vi "WMI Get Battery Status.vi"() -> (0 "Discharging?":bool, 1 "estRT":i32, 2 "estCharge":u8, 3 "Status":string)   [LabVIEW 2013]
doc: "Use the WMI to return the battery status, including the estimated battery life remaining and the time until the battery is fully discharged.\n\nInformation regarding the WMI battery class may be found at http://msdn.microsoft.com/en-us/library/aa394074%28v=vs.85%29.aspx."
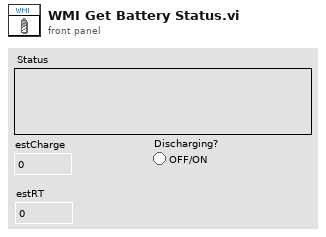
[diagram p1: front panel]
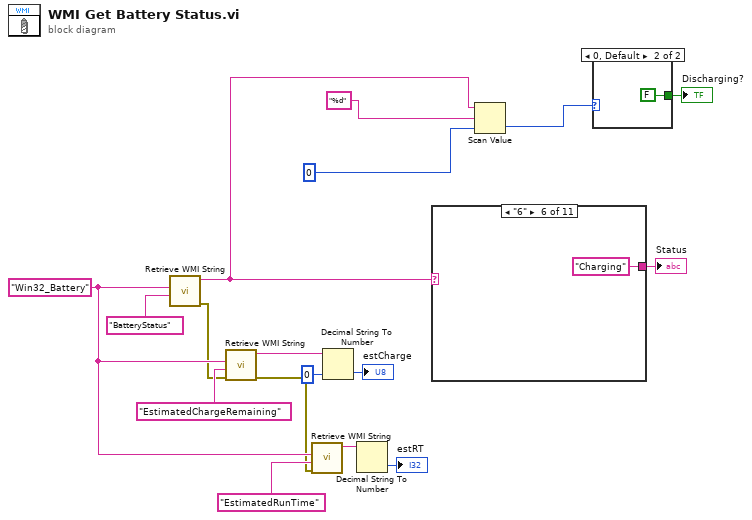
[diagram p0: block diagram]
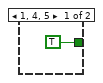
[diagram p2: hidden frame]
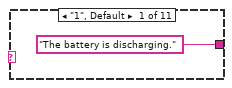
[diagram p3: hidden frame]
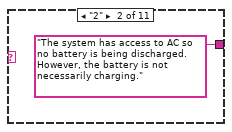
[diagram p4: hidden frame]
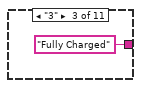
[diagram p5: hidden frame]
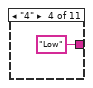
[diagram p6: hidden frame]
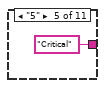
[diagram p7: hidden frame]
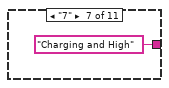
[diagram p8: hidden frame]
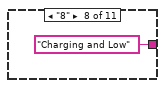
[diagram p9: hidden frame]
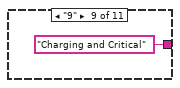
[diagram p10: hidden frame]
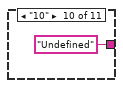
[diagram p11: hidden frame]
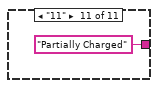
[diagram p12: hidden frame]
diagram:
  w15 = "Win32_Battery" ("wmiClass")
  n1 = call "Retrieve WMI String.vi"("wmiProperty"="BatteryStatus", "wmiClass"=w15) -> ("Error Out"=w7:errorcluster, "LastValue"=w2:string)  [unwired: 7 in, 1 out]
  n2 = call "Retrieve WMI String.vi"("error in"=w7, "wmiProperty"="EstimatedChargeRemaining", "wmiClass"=w15) -> ("Error Out"=w8:errorcluster, "LastValue"=w11:string)  [unwired: 6 in, 1 out]
  n3 = call "Retrieve WMI String.vi"("error in"=w8, "wmiProperty"="EstimatedRunTime", "wmiClass"=w15) -> ("LastValue"=w13:string)  [unwired: 6 in, 2 out]
  n4 = Decimal String To Number(string=w11, default (0L)=u8 0 ("default (0 I32)")) -> (number=→"estCharge":u8)  [unwired: 1 in, 1 out]
  n5 = Decimal String To Number(string=w13) -> (number=→"estRT":i32)  [unwired: 2 in, 1 out]
  n6 = case shown="\"6\"" w2 {
    tunnel: ["The battery is discharging." "The system has access to AC so no battery is being discharged. However, the battery is not necessarily charging." "Fully Charged" "Low" "Critical" "Charging" "Charging and High" "Charging and Low" "Charging and Critical" "Undefined" "Partially Charged"] -> w9
    frame "1", Default {
    }
    frame "2" {
    }
    frame "3" {
    }
    frame "4" {
    }
    frame "5" {
    }
    frame "6" {
    }
    frame "7" {
    }
    frame "8" {
    }
    frame "9" {
    }
    frame "10" {
    }
    frame "11" {
    }
  }
  "Status" <- w9
  n7 = Scan Value(string=w2, format string="%d", default (0 dbl)=u8 0 ("estBattLeft 2")) -> (value=w3:u8)  [unwired: 1 out]
  n8 = case shown="0, Default" w3 {
    tunnel: [TRUE FALSE] -> w1
    frame 1, 4, 5 {
    }
    frame 0, Default {
    }
  }
  "Discharging?" <- w1
